vi "New-View.vi"(8 "error in (no error)":errorcluster) -> (0 "error out":errorcluster, 3 "View out":refnum<class "View.lvclass">)   [LabVIEW 2024, in "GLF.lvlib" / "View.lvclass"]
uses:
  View.lvclass
  View.lvclass/View.ctl
  IAmGLF/IAmGLF.lvclass
  C:/Users/Thomas/Documents/Projects/GLF/Sources/GLF/IUseDVRHandler/IUseDVRHandler.lvclass
  C:/Users/Thomas/Documents/Projects/GLF/Sources/GLF/IAmGLF/IAmGLF.lvclass
  C:/Users/Thomas/Documents/Projects/GLF/Sources/GLF/View/View.lvclass
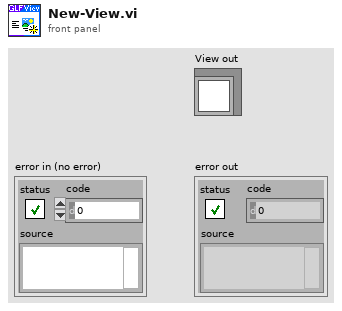
[diagram p1: front panel]
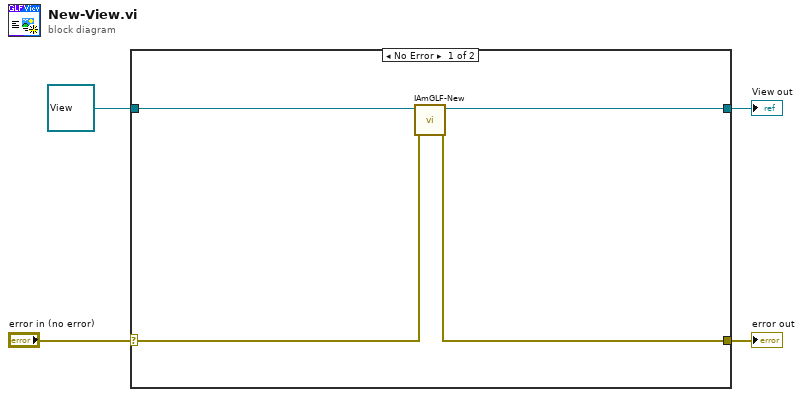
[diagram p0: block diagram]
diagram:
  n1 = case shown="No Error" "error in (no error)" {
    selector: "error in (no error)" -> [w6 w10]
    tunnel: [w5 w10] -> w3
    tunnel: [w7 w9] -> w1
    tunnel: refnum<class "View.lvclass"> refnum ("View in") -> [w8 w9]
    frame No Error {
      n2 = call "IAmGLF-New.vi"("error in (no error)"=w6, "IAmGLF in"=w8) -> ("error out"=w5:errorcluster, "IAmGLF out"=w7:refnum<class "View.lvclass">)  [unwired: 8 in]
    }
    frame Error {
    }
  }
  "error out" <- w3
  "View out" <- w1
